vi "RefreshUI.vi"(8 "error in (no error)":errorcluster, 11 "View in":refnum<class "View.lvclass">) -> (0 "error out":errorcluster, 3 "View out":refnum<class "View.lvclass">)   [LabVIEW 2020, in "View.lvclass"]
uses:
  View.lvclass
  View.lvclass/View.ctl
  Controller/Controller.lvclass
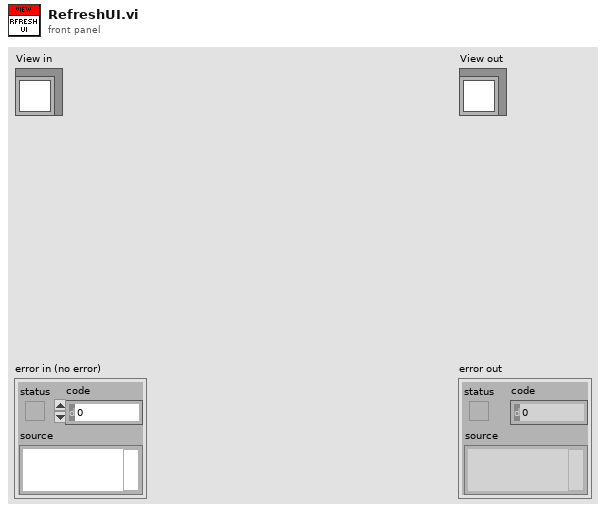
[diagram p1: front panel]
types:
  T1 = cluster{"View:Integer":refnum<vi>, "Model:Integer":refnum<vi>}
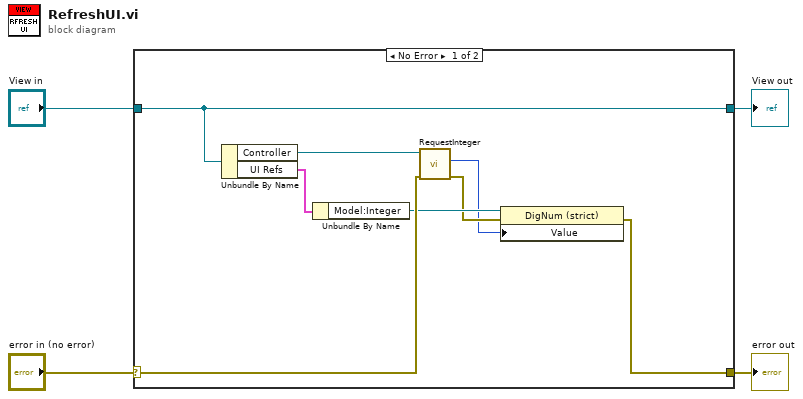
[diagram p0: block diagram]
diagram:
  n1 = case shown="No Error" "error in (no error)" {
    selector: "error in (no error)" -> [w10 w14]
    tunnel: [w5 w14] -> w3
    tunnel: [w12 w13] -> w1
    tunnel: "View in" -> [w12 w13]
    frame No Error {
      n2 = Unbundle By Name(w12) -> ("Controller"=w11:refnum<class "Controller.lvclass">, "UI Refs"=w9:T1)
      n3 = Unbundle By Name(w9) -> ("Model:Integer"=w8:refnum<vi>)
      n4 = call "RequestInteger.vi"("error in (no error)"=w10, "Controller in"=w11) -> ("error out"=w7:errorcluster, "Integer"=w6:i32)  [unwired: 7 in, 1 out]
      n5 = property class="DigNum (strict)"(reference=w8, error in=w7, "Value"=w6) -> (error out=w5:errorcluster)  [unwired: 1 out]
    }
    frame Error {
    }
  }
  "error out" <- w3
  "View out" <- w1
